vi "Send Request.vi"(8 "error in (no error)":errorcluster, 11 "Request-Reply Reference":refnum<data-value>) -> (0 "error out":errorcluster)   [LabVIEW 2018, in "Templates.lvlib"]
uses:
  Templates.lvlib
  Actor/Actor.lvclass
  Actor/Stop.ctl
  Actor/Did Stop.ctl
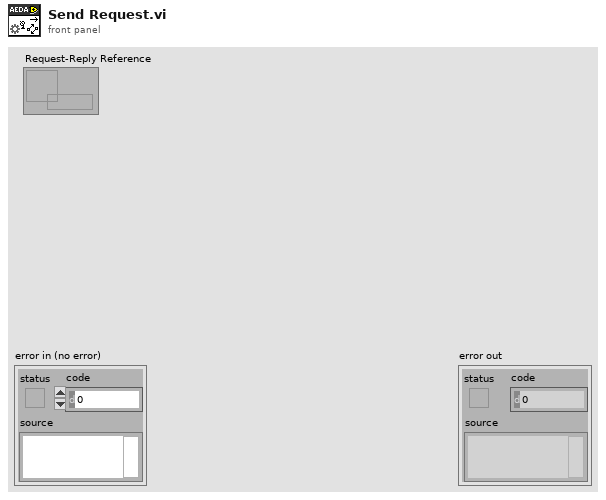
[diagram p1: front panel]
types:
  T1 = typedef "Templates.lvlib/Actor.lvclass/Stop.ctl" = cluster{"Type":enum16{"Normal", "Emergency"}}
  T2 = cluster{"Stop":refnum<user-event>, "cluster":cluster{"Stopped":refnum<user-event>, "Stop":T1}}
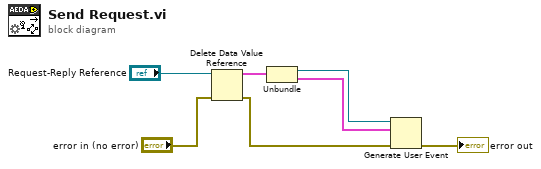
[diagram p0: block diagram]
diagram:
  n1 = Delete Data Value Reference(data value reference="Request-Reply Reference", error in="error in (no error)") -> (data value=w3:T2, error out=w5:errorcluster)
  n2 = Unbundle(w3) -> ("Stop"=w2:refnum<user-event>, "cluster"=w1:cluster{"Stopped":refnum<user-event>, "Stop":T1})
  n3 = Generate User Event(user event=w2, event data cluster=w1, error in=w5) -> (error out=→"error out":errorcluster)  [unwired: 1 in, 1 out]
